vi "BalanceSizeArray.vi"(5 "Max Stroke":i32, 6 "MaxForce":bool, 7 "Min Stroke":i32, 8 "Analog RW In":T1, 9 "CountDeleteIn":i32, 10 "TotalSizeIn":i32, 11 "Analog FW In":T1) -> (0 "Analog RW Out":T1, 3 "Analog FW Out":T1)   [LabVIEW 2017]
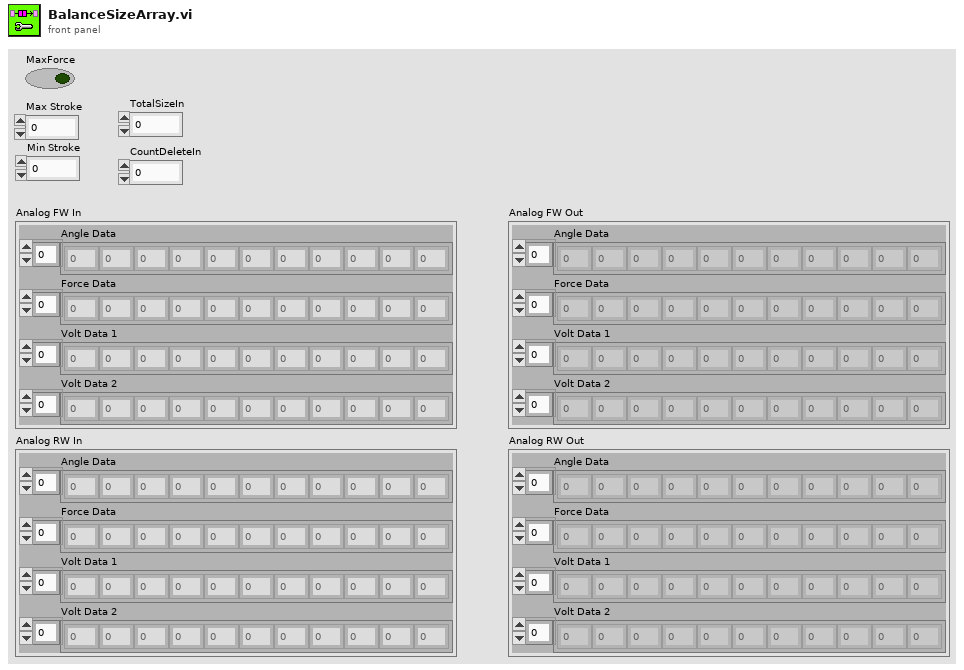
[diagram p1: front panel]
types:
  T1 = cluster{"Angle Data":dbl[], "Force Data":dbl[], "Volt Data 1":dbl[], "Volt Data 2":dbl[]}
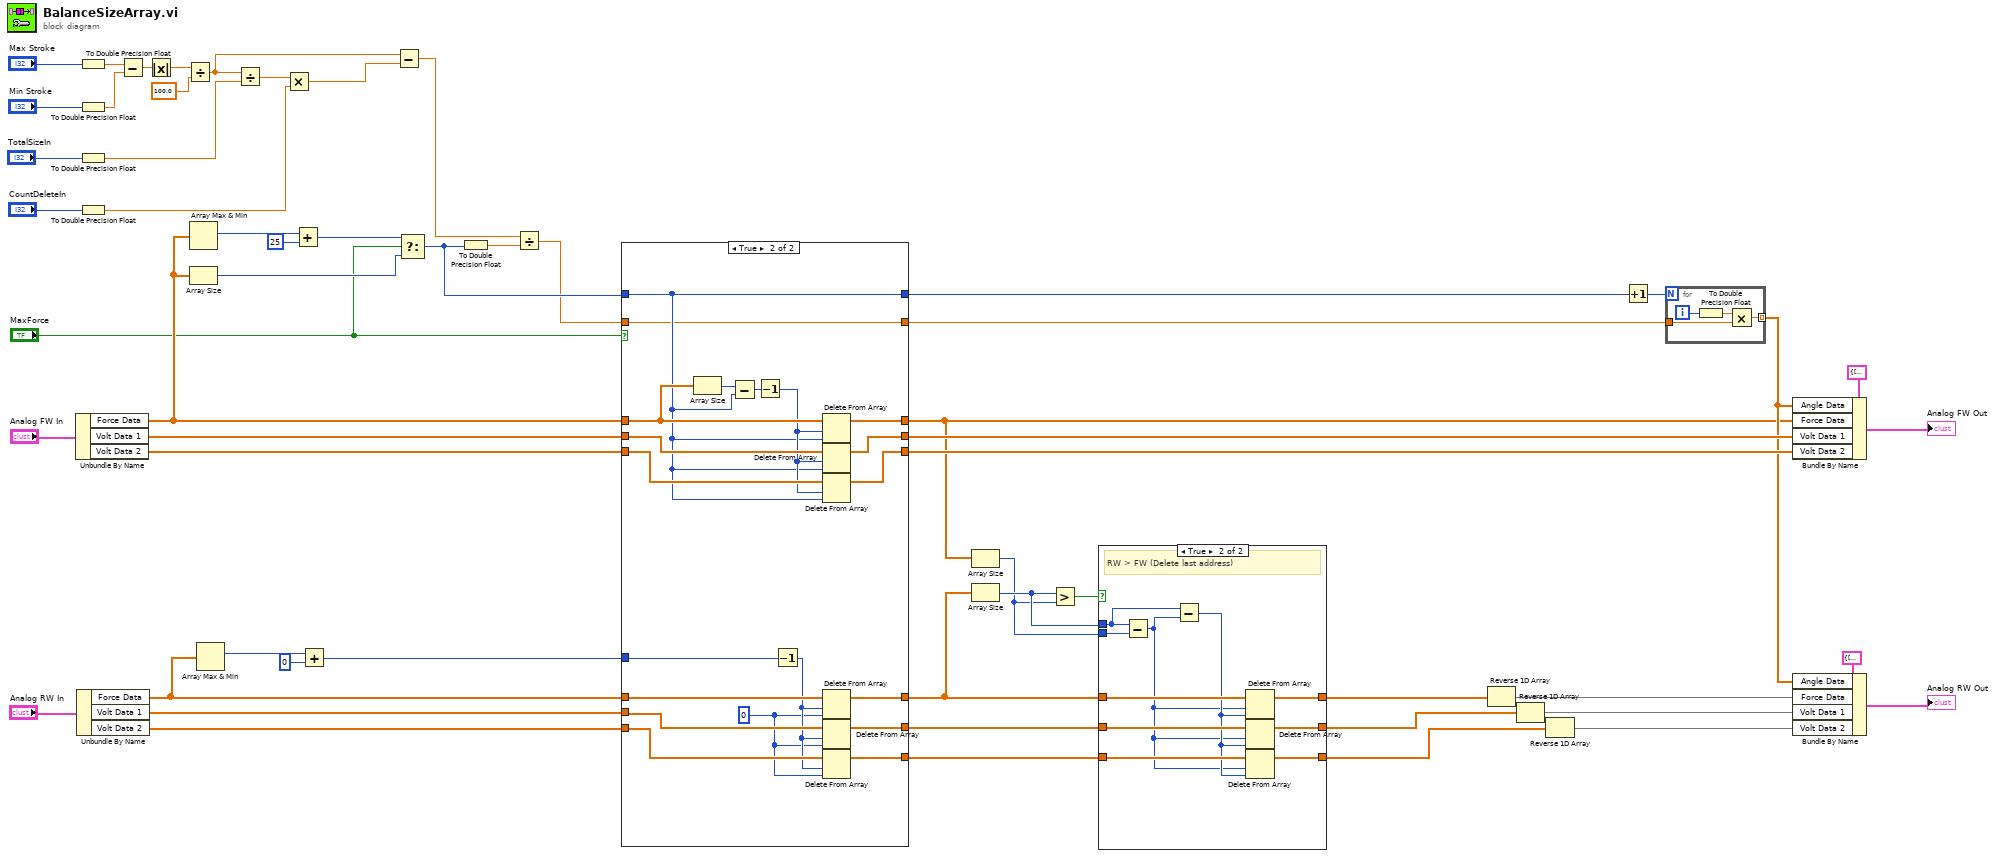
[diagram p0: block diagram]
diagram:
  n1 = Unbundle By Name("Analog FW In") -> ("Force Data"=w39:dbl[], "Volt Data 1"=w38:dbl[], "Volt Data 2"=w37:dbl[])
  n2 = Unbundle By Name("Analog RW In") -> ("Force Data"=w15:dbl[], "Volt Data 1"=w34:dbl[], "Volt Data 2"=w33:dbl[])
  n3 = To Double Precision Float(number="Max Stroke") -> (double precision float=w51:dbl)
  n4 = To Double Precision Float(number="Min Stroke") -> (double precision float=w50:dbl)
  n5 = To Double Precision Float(number="TotalSizeIn") -> (double precision float=w28:dbl)
  n6 = To Double Precision Float(number="CountDeleteIn") -> (double precision float=w22:dbl)
  n7 = Subtract(x=w51, y=w50) -> (x-y=w47:dbl)
  n8 = Absolute Value(x=w47) -> (abs(x)=w49:dbl)
  n9 = Divide(x=w49, y=100.0) -> (x/y=w21:dbl)
  n10 = Array Max & Min(array=w39) -> (max index (indices)=w43:i32)  [unwired: 3 out]
  n11 = Array Size(array=w39) -> (size(s)=w40:i32)
  n12 = Array Max & Min(array=w15) -> (max index (indices)=w16:i32)  [unwired: 3 out]
  n13 = Divide(x=w21, y=w28) -> (x/y=w24:dbl)
  n14 = Multiply(x=w24, y=w22) -> (x*y=w20:dbl)
  n15 = Add(x=w43, y=25) -> (x+y=w42:i32)
  n16 = Add(x=w16, y=0) -> (x+y=w11:i32)
  n17 = Subtract(x=w21, y=w20) -> (x-y=w13:dbl)
  n18 = Select(t=w42, s="MaxForce", f=w40) -> (s? t:f=w27:i32)
  n19 = To Double Precision Float(number=w27) -> (double precision float=w44:dbl)
  n20 = Divide(x=w13, y=w44) -> (x/y=w25:dbl)
  n21 = case shown="True" "MaxForce" {
    tunnel: w39 -> [w65 w85]
    tunnel: w38 -> [w64 w83]
    tunnel: w37 -> [w63 w82]
    tunnel: [w65 w81] -> w10
    tunnel: [w64 w80] -> w36
    tunnel: [w63 w79] -> w35
    tunnel: [w62 w77] -> w6
    tunnel: w15 -> [w62 w71]
    tunnel: [w61 w74] -> w4
    tunnel: w34 -> [w61 w76]
    tunnel: [w60 w73] -> w3
    tunnel: w33 -> [w60 w75]
    tunnel: w27 -> [w59 w69]
    tunnel: [w59 w69] -> w19
    tunnel: [w58 w68] -> w26
    tunnel: w25 -> [w58 w68]
    tunnel: w11 -> [_ w66]
    frame False {
    }
    frame True {
      w67 = 0 ("index")
      n22 = Array Size(array=w85) -> (size(s)=w84:i32)
      n23 = Subtract(x=w84, y=w69) -> (x-y=w78:i32)
      n24 = Decrement(x=w78) -> (x-1=w72:i32)
      n25 = Decrement(x=w66) -> (x-1=w70:i32)
      n26 = Delete From Array(array=w85, length=w72, index=w69) -> (array with subset deleted=w81:dbl[])  [unwired: 1 out]
      n27 = Delete From Array(array=w83, length=w72, index=w69) -> (array with subset deleted=w80:dbl[])  [unwired: 1 out]
      n28 = Delete From Array(array=w82, length=w72, index=w69) -> (array with subset deleted=w79:dbl[])  [unwired: 1 out]
      n29 = Delete From Array(array=w71, length=w70, index=w67) -> (array with subset deleted=w77:dbl[])  [unwired: 1 out]
      n30 = Delete From Array(array=w76, length=w70, index=w67) -> (array with subset deleted=w74:dbl[])  [unwired: 1 out]
      n31 = Delete From Array(array=w75, length=w70, index=w67) -> (array with subset deleted=w73:dbl[])  [unwired: 1 out]
    }
  }
  n32 = Array Size(array=w10) -> (size(s)=w7:i32)
  n33 = Array Size(array=w6) -> (size(s)=w8:i32)
  n34 = Greater?(x=w8, y=w7) -> (0:w9:bool)
  n35 = case shown="True" w9 {
    tunnel: w8 -> [_ w91]
    tunnel: w7 -> [_ w98]
    tunnel: w6 -> [w88 w97]
    tunnel: [w88 w96] -> w5
    tunnel: w4 -> [w87 w95]
    tunnel: w3 -> [w86 w94]
    tunnel: [w87 w93] -> w2
    tunnel: [w86 w92] -> w1
    frame False {
    }
    frame True {
      # "RW > FW (Delete last address)"
      n36 = Subtract(x=w91, y=w98) -> (x-y=w89:i32)
      n37 = Subtract(x=w91, y=w89) -> (x-y=w90:i32)
      n38 = Delete From Array(array=w97, length=w89, index=w90) -> (array with subset deleted=w96:dbl[])  [unwired: 1 out]
      n39 = Delete From Array(array=w95, length=w89, index=w90) -> (array with subset deleted=w93:dbl[])  [unwired: 1 out]
      n40 = Delete From Array(array=w94, length=w89, index=w90) -> (array with subset deleted=w92:dbl[])  [unwired: 1 out]
    }
  }
  n41 = Reverse 1D Array(array=w5) -> (reversed array=w30:dbl[])
  n42 = Reverse 1D Array(array=w2) -> (reversed array=w32:dbl[])
  n43 = Reverse 1D Array(array=w1) -> (reversed array=w31:dbl[])
  n44 = Increment(x=w19) -> (x+1=w18:i32)
  n45 = for {
    N: w18 -> [_]
    tunnel: w26 -> [w102]
    tunnel: [w99] -> w12 mode=indexing
    i -> [w100]
    n46 = To Double Precision Float(number=w100) -> (double precision float=w101:dbl)
    n47 = Multiply(x=w101, y=w102) -> (x*y=w99:dbl)
  }
  n48 = Bundle By Name(cluster=T1 {"Angle Data"=[], "Force Data"=[], "Volt Data 1"=[], "Volt Data 2"=[]} ("Analog FW Out"), "Angle Data"=w12, "Force Data"=w10, "Volt Data 1"=w36, "Volt Data 2"=w35) -> (→"Analog FW Out":T1)
  n49 = Bundle By Name(cluster=T1 {"Angle Data"=[], "Force Data"=[], "Volt Data 1"=[], "Volt Data 2"=[]} ("Analog FW Out"), "Angle Data"=w12, "Force Data"=w30, "Volt Data 1"=w32, "Volt Data 2"=w31) -> (→"Analog RW Out":T1)
